vi "Mapping v10.2.2.vi"(5 "Simulate Spectra":bool, 7 "Simulate Drive":bool, 11 "Input Parameters":T9={"CCD3000 Connection"={"Comm Interface"=1, "BUS"=0, "Address"=5, "Com Port"=1}, "Drive Connection Settings"={"Objective GPIB-Port"=4, "Stage GPIB-Port"=4, "Drive Selector"=0, "Drive Velocity (V/s)"=5.0}, "ITC503 Current Values"={"ITC503 Heater"=0.0, "ITC503 Temperature"=0.0, "ITC503 P"=0.0, "ITC503 I"=0.0, "ITC503 D"=0.0, "ITC503 Setpoint"=0.0, "ITC503 Gradient"=0.0, "ITC503 Heater Auto"=FALSE, "ITC503 PID Auto"=FALSE}, "Wavelengths (nm)"=[], "Drive Current Values"={"Voltages"={"Drive X Voltage"=0.0, "Drive Y Voltage"=0.0, "Drive Z Voltage"=0.0}, "Position"={"Drive X Position"=0.0, "Drive Y Position"=0.0, "Drive Z Position"=0.0}}, "iHR Current Values"={"iHR 550 Front Entrance"=0.0, "iHR550 Side Exit"=0.0, "iHR550 Wavelength"=897.9988, "iHR550 Exit Mirror"=2, "iHR550 Grating"="1", "Grating Index"=1}, "Spectra Settings"={"Integration Time"=1.0, "Repetitions"=1, "Mapping Spectra"=TRUE}, "CCD3500 Temperature"=0.0, "Simulate Drive"=FALSE, "Simulate Spectra"=FALSE} {"CCD3500 Temperature" min=10.0 max=160.0 step=0.1 format="%.1f"; "Spectra Settings"."Repetitions" min=1 max=100 step=1; "Spectra Settings"."Integration Time" min=0.5 max=6000.0 step=1.0 format="%.1f"; "iHR Current Values"."iHR550 Exit Mirror" items=["EntranceMirror", "ExitMirror", "Front", "Side"]; "Drive Current Values"."Position"."Drive Z Position" min=-273.0 max=300000.0 step=0.0001 format="%.1f"; "Drive Current Values"."Position"."Drive Y Position" min=-273.0 max=300000.0 step=0.0001 format="%.1f"; "Drive Current Values"."Position"."Drive X Position" min=-273.0 max=300000.0 step=0.0001 format="%.1f"; "Drive Current Values"."Voltages"."Drive Z Voltage" min=-273.0 max=300000.0 step=0.0001 format="%.1f"; "Drive Current Values"."Voltages"."Drive Y Voltage" min=-273.0 max=300000.0 step=0.0001 format="%.1f"; "Drive Current Values"."Voltages"."Drive X Voltage" min=-273.0 max=300000.0 step=0.0001 format="%.1f"; "ITC503 Current Values"."ITC503 Gradient" format="%.2f"; "ITC503 Current Values"."ITC503 Setpoint" min=-273.0 max=300000.0 step=0.0001 format="%.1f"; "ITC503 Current Values"."ITC503 I" format="%_1f"; "ITC503 Current Values"."ITC503 P" format="%_1f"; "ITC503 Current Values"."ITC503 Temperature" min=0.0 max=1645.0 step=1e-05 format="%.2f"; "ITC503 Current Values"."ITC503 Heater" min=0.0 max=100.0 step=0.01 scale=0.0..100.0; "Drive Connection Settings"."Drive Velocity (V/s)" min=10.0 max=160.0 step=0.1 format="%.1f"; "Drive Connection Settings"."Drive Selector" items=["Obj.", "Stage"]; "Drive Connection Settings"."Stage GPIB-Port" min=1 max=20 step=1 format="%#.0f"; "Drive Connection Settings"."Objective GPIB-Port" min=1 max=20 step=1 format="%#.0f"; "CCD3000 Connection"."Comm Interface" items=["RS 232", "GPIB"]}) -> ()   [LabVIEW 2010]
uses:
  ESA-C/TypeDefs/ESA-C Connection Settings.ctl
  TypeDefs/Mapping Spectra Params.ctl
  TypeDefs/Mapping Drive Params.ctl
  ESA-C/TypeDefs/ESA-C Set Positions.ctl
  ESA-C/TypeDefs/ESA-C Current Values.ctl
  iHR550/TypeDefs/iHR Current Values.ctl
  ITC503/TypeDefs/ITC503 Current Values.ctl
  drivers/Horiba Spectrum One 3000V/Lib/CCD_command.llb/Comm Params.ctl
  <vilib>/Utility/miscctls.llb/LVPointTypeDef.ctl
panel:
  in  "Pause":bool
  out "Current Position":T1 {"Position"."Drive Z Position" min=-273.0 max=300000.0 step=0.0001 format="%.1f"; "Position"."Drive Y Position" min=-273.0 max=300000.0 step=0.0001 format="%.1f"; "Position"."Drive X Position" min=-273.0 max=300000.0 step=0.0001 format="%.1f"; "Voltages"."Drive Z Voltage" min=-273.0 max=300000.0 step=0.0001 format="%.1f"; "Voltages"."Drive Y Voltage" min=-273.0 max=300000.0 step=0.0001 format="%.1f"; "Voltages"."Drive X Voltage" min=-273.0 max=300000.0 step=0.0001 format="%.1f"}
  out "Target Position":T2={"Drive X Set"=10.0, "Drive Y Set"=10.0, "Drive Z Set"=10.0} {"Drive X Set" min=10.0 max=160.0 step=0.1 format="%.1f"; "Drive Z Set" min=10.0 max=160.0 step=0.1 format="%.1f"; "Drive Y Set" min=10.0 max=160.0 step=0.1 format="%.1f"}
  out "Progress":u8(slide) max=10 scale=0.0..100.0
  out "Objective Running":bool caption="Obj."
  out "CCD Running":bool caption="CCD"
  in  "Save Map":bool
  in  "CCD3000 Current Rep.":string="0/0"
  in  "Spectra Params":T3={"Integration Time"=10.0, "Repetitions"=10, "Mapping Spectra"=TRUE} {"Repetitions" min=1 max=100 step=1; "Integration Time" min=0.5 max=6000.0 step=1.0 format="%.1f"}
  in  "Drive Settings":T4={"Objective GPIB-Port"=4, "Stage GPIB-Port"=4, "Drive Selector"=0, "Drive Velocity (V/s)"=5.0} {"Drive Velocity (V/s)" min=10.0 max=160.0 step=0.1 format="%.1f"; "Drive Selector" items=["Obj.", "Stage"]; "Stage GPIB-Port" min=1 max=20 step=1 format="%#.0f"; "Objective GPIB-Port" min=1 max=20 step=1 format="%#.0f"}
  in  "Z Position":dbl caption="Z (µm)" min=0.0 max=100.0 step=0.1 format="%.1f"
  in  "Mapping Params":T5={"X Start Position"=0.0, "X Stop Position"=10.0, "Y Start Position"=0.0, "Y Stop Position"=10.0, "Step Size"=1.0} {"Step Size" min=0.1 max=30.0 step=0.1 format="%.1f"; "Y Stop Position" min=0.0 max=30.0 step=0.1 format="%.1f"; "Y Start Position" min=0.0 max=30.0 step=0.1 format="%.1f"; "X Stop Position" min=0.0 max=30.0 step=0.1 format="%.1f"; "X Start Position" min=0.0 max=30.0 step=0.1 format="%.1f"}
  in  "Exit":bool
  out "Measuring":bool
  in  "Start":bool
  out "Filename":string
  out "Full Data":dbl[][](array[numeric])
  in  "CCD3500V Connection":T10={"Comm Interface"=1, "BUS"=0, "Address"=5, "Com Port"=0}
  out "Live Data":dbl[][](array[numeric])
  in  "ITC503 Current Values":T7 {"ITC503 Gradient" format="%.2f"; "ITC503 Setpoint" min=-273.0 max=300000.0 step=0.0001 format="%.1f"; "ITC503 I" format="%_1f"; "ITC503 P" format="%_1f"; "ITC503 Temperature" min=0.0 max=1645.0 step=1e-05 format="%.2f"; "ITC503 Heater" min=0.0 max=100.0 step=0.01 scale=0.0..100.0}
  in  "iHR Current Values":T8={"iHR 550 Front Entrance"=0.0, "iHR550 Side Exit"=0.0, "iHR550 Wavelength"=897.9988, "iHR550 Exit Mirror"=2, "iHR550 Grating"="1", "Grating Index"=1} {"iHR550 Exit Mirror" items=["EntranceMirror", "ExitMirror", "Front", "Side"]}
  in  "CCD3500 Temperature":dbl caption="Temp. (°C)" min=10.0 max=160.0 step=0.1 format="%.1f"
  in  "Wavelengths (nm)":dbl[](array[numeric])
  # "Status"
  # "Active"
  # "Target"
  # "Current"
  # "Spectral"
  # "Spectral / Video Mapping"
  # "Parameters"
  # "GPIB"
  # "Mapping"
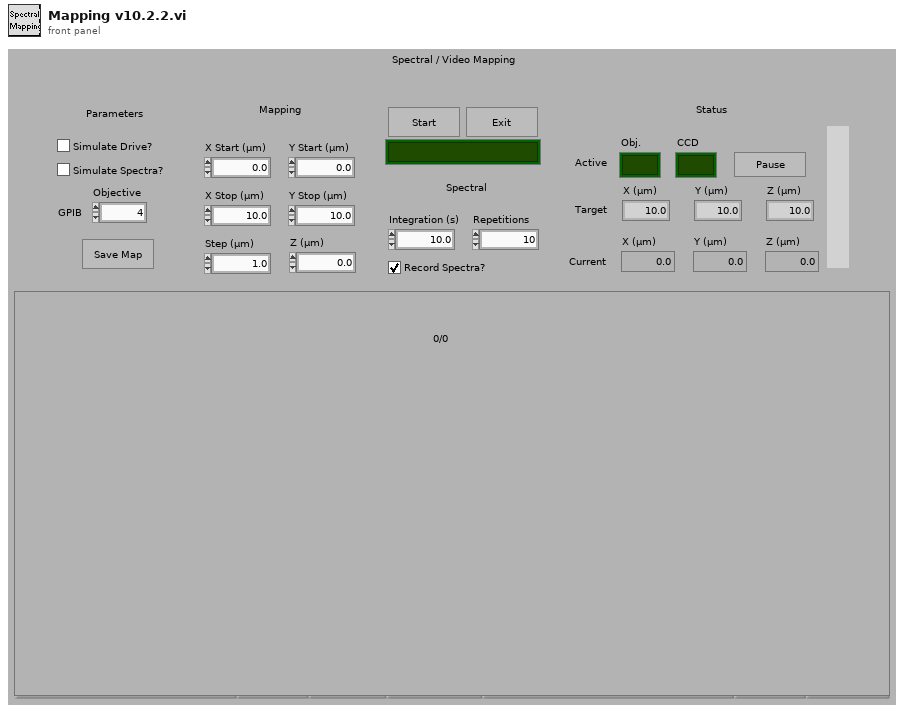
[diagram p1: front panel]
types:
  T1 = typedef "ESA-C Current Values.ctl" = cluster{"Voltages":cluster{"Drive X Voltage":dbl, "Drive Y Voltage":dbl, "Drive Z Voltage":dbl}, "Position":cluster{"Drive X Position":dbl, "Drive Y Position":dbl, "Drive Z Position":dbl}}
  T2 = typedef "ESA-C Set Positions.ctl" = cluster{"Drive X Set":dbl, "Drive Y Set":dbl, "Drive Z Set":dbl}
  T3 = typedef "Mapping Spectra Params.ctl" = cluster{"Integration Time":dbl, "Repetitions":u16, "Mapping Spectra":bool}
  T4 = typedef "ESA-C Connection Settings.ctl" = cluster{"Objective GPIB-Port":i32, "Stage GPIB-Port":i32, "Drive Selector":u16, "Drive Velocity (V/s)":dbl}
  T5 = typedef "Mapping Drive Params.ctl" = cluster{"X Start Position":dbl, "X Stop Position":dbl, "Y Start Position":dbl, "Y Stop Position":dbl, "Step Size":dbl}
  T6 = typedef "Comm Params.ctl" = cluster{"Comm Interface":u16, "BUS":i16, "Address":i16, "Com Port":i32}
  T7 = typedef "ITC503 Current Values.ctl" = cluster{"ITC503 Heater":dbl, "ITC503 Temperature":dbl, "ITC503 P":dbl, "ITC503 I":dbl, "ITC503 D":dbl, "ITC503 Setpoint":dbl, "ITC503 Gradient":dbl, "ITC503 Heater Auto":bool, "ITC503 PID Auto":bool}
  T8 = typedef "iHR Current Values.ctl" = cluster{"iHR 550 Front Entrance":dbl, "iHR550 Side Exit":dbl, "iHR550 Wavelength":dbl, "iHR550 Exit Mirror":i32, "iHR550 Grating":string, "Grating Index":i32}
  T9 = cluster{"CCD3000 Connection":T6, "Drive Connection Settings":T4, "ITC503 Current Values":T7, "Wavelengths (nm)":dbl[], "Drive Current Values":T1, "iHR Current Values":T8, "Spectra Settings":T3, "CCD3500 Temperature":dbl, "Simulate Drive":bool, "Simulate Spectra":bool}
  T10 = cluster{"Comm Interface":u16, "BUS":i16, "Address":i16, "Com Port":i32}
  T11 = cluster{"CCD3000 Connection":T6, "Drive Connection Settings":T4, "ITC503 Current Values":T7, "Wavelengths (nm)":dbl[], "Drive Current Values":T1, "iHR Current Values":T8, "Spectra Settings":T3, "CCD3500 Temperature":dbl, "Simulate Drive 2":bool, "Simulate Spectra 2":bool}
  T12 = typedef "LVPointTypeDef.ctl" = cluster{"Horizontal":i16, "Vertical":i16}
  T13 = typedef "NPC3SG Set Positions.ctl" = cluster{"Drive X Set":dbl, "Drive Y Set":dbl, "Drive Z Set":dbl}
  T14 = cluster{"Intensities":dbl[], "Wavelengths":dbl[]}[]
  T15 = cluster{"Intensities":dbl[], "Wavelengths":dbl[]}
  T16 = enum32{"invalid app kind", "Development System", "Run Time System", "Student Edition", "Embedded LabVIEW", "Evaluation", "Custom"}
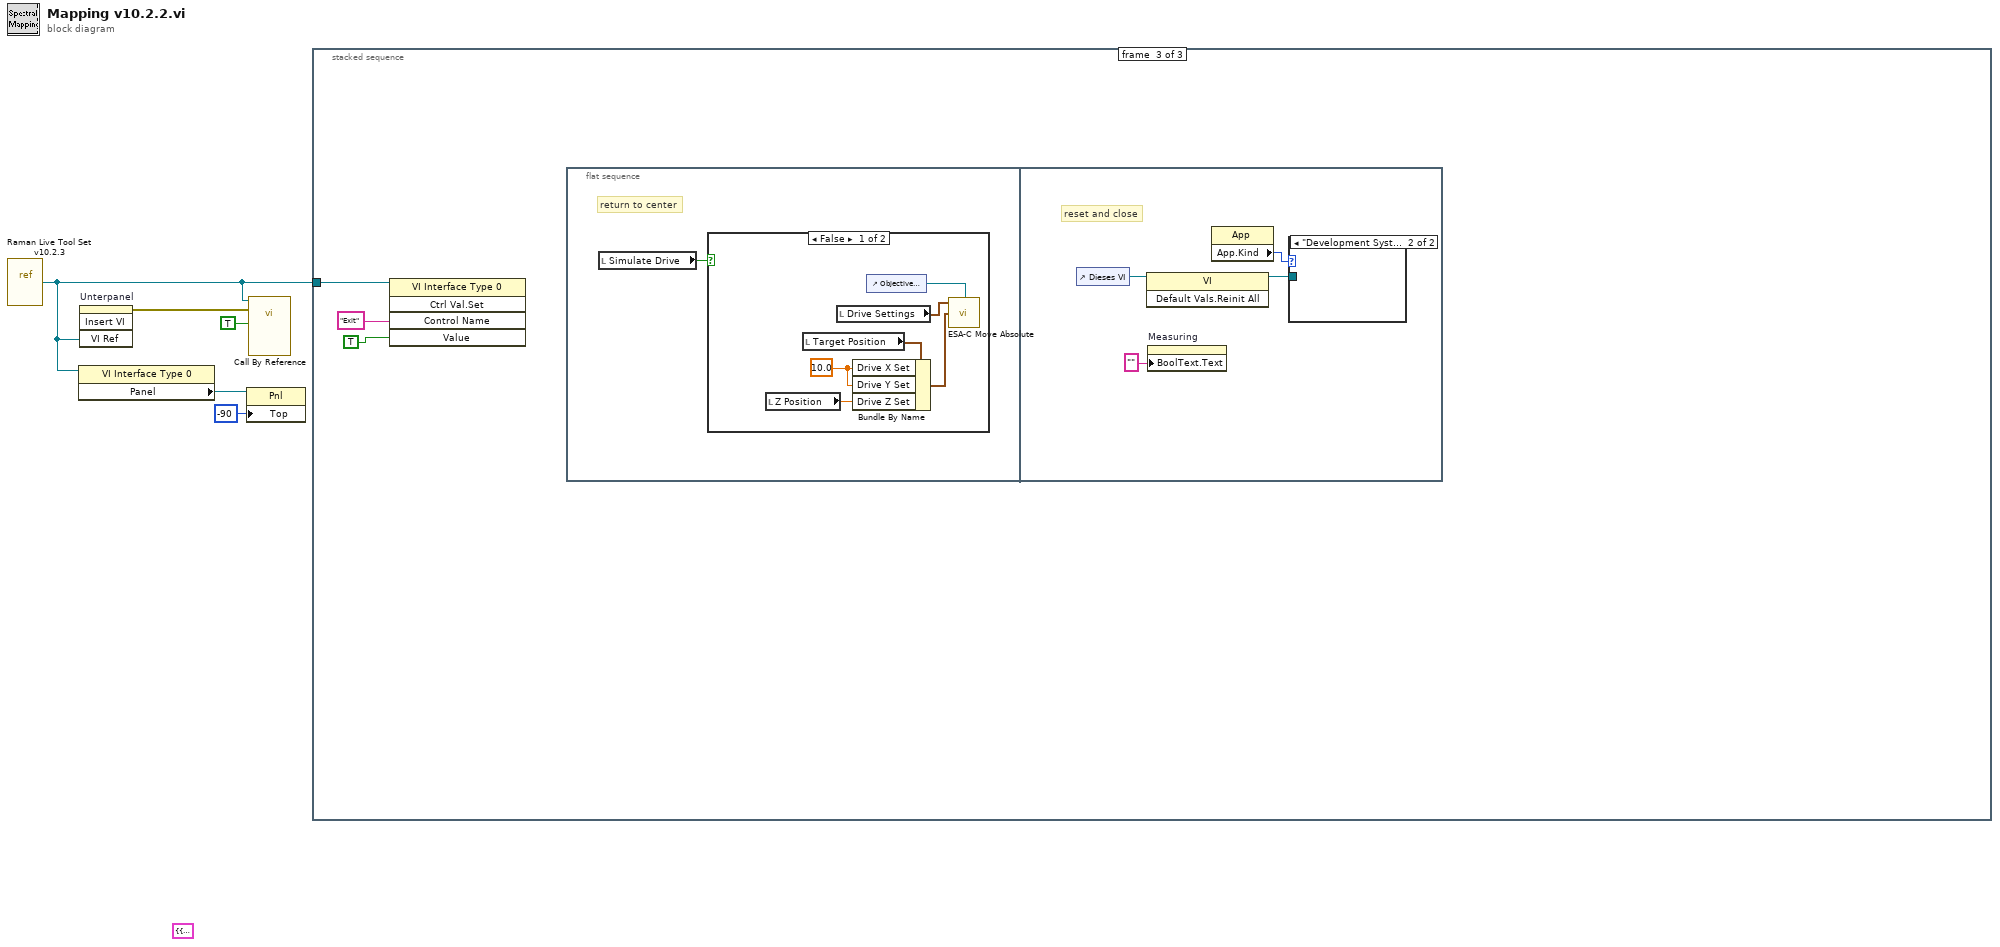
[diagram p0: block diagram]
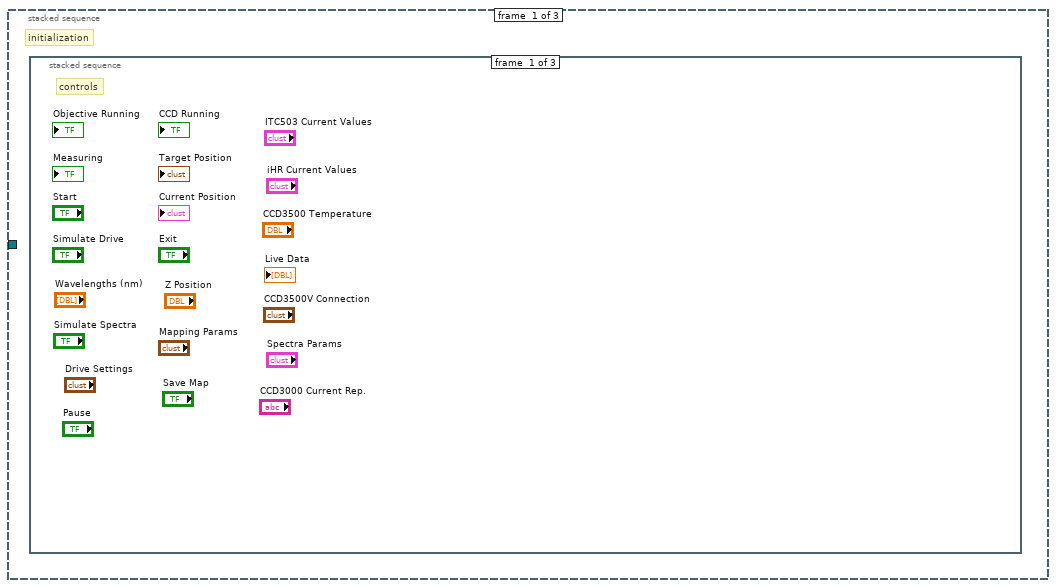
[diagram p2: hidden frame]
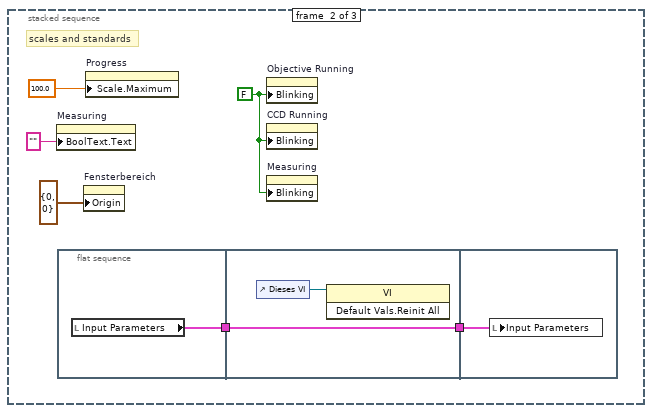
[diagram p3: hidden frame]
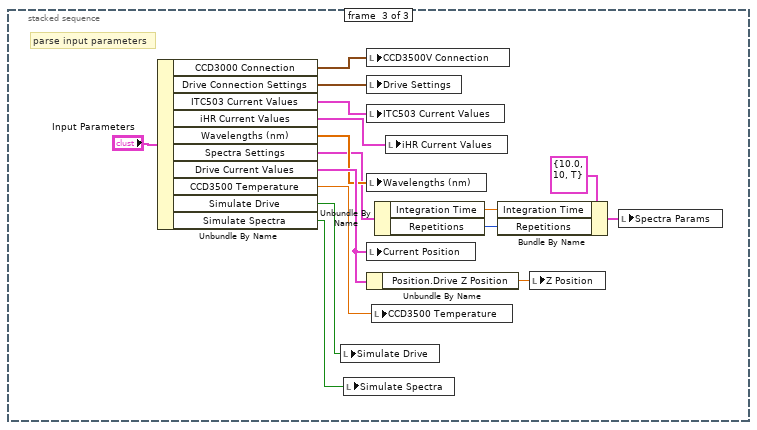
[diagram p4: hidden frame]
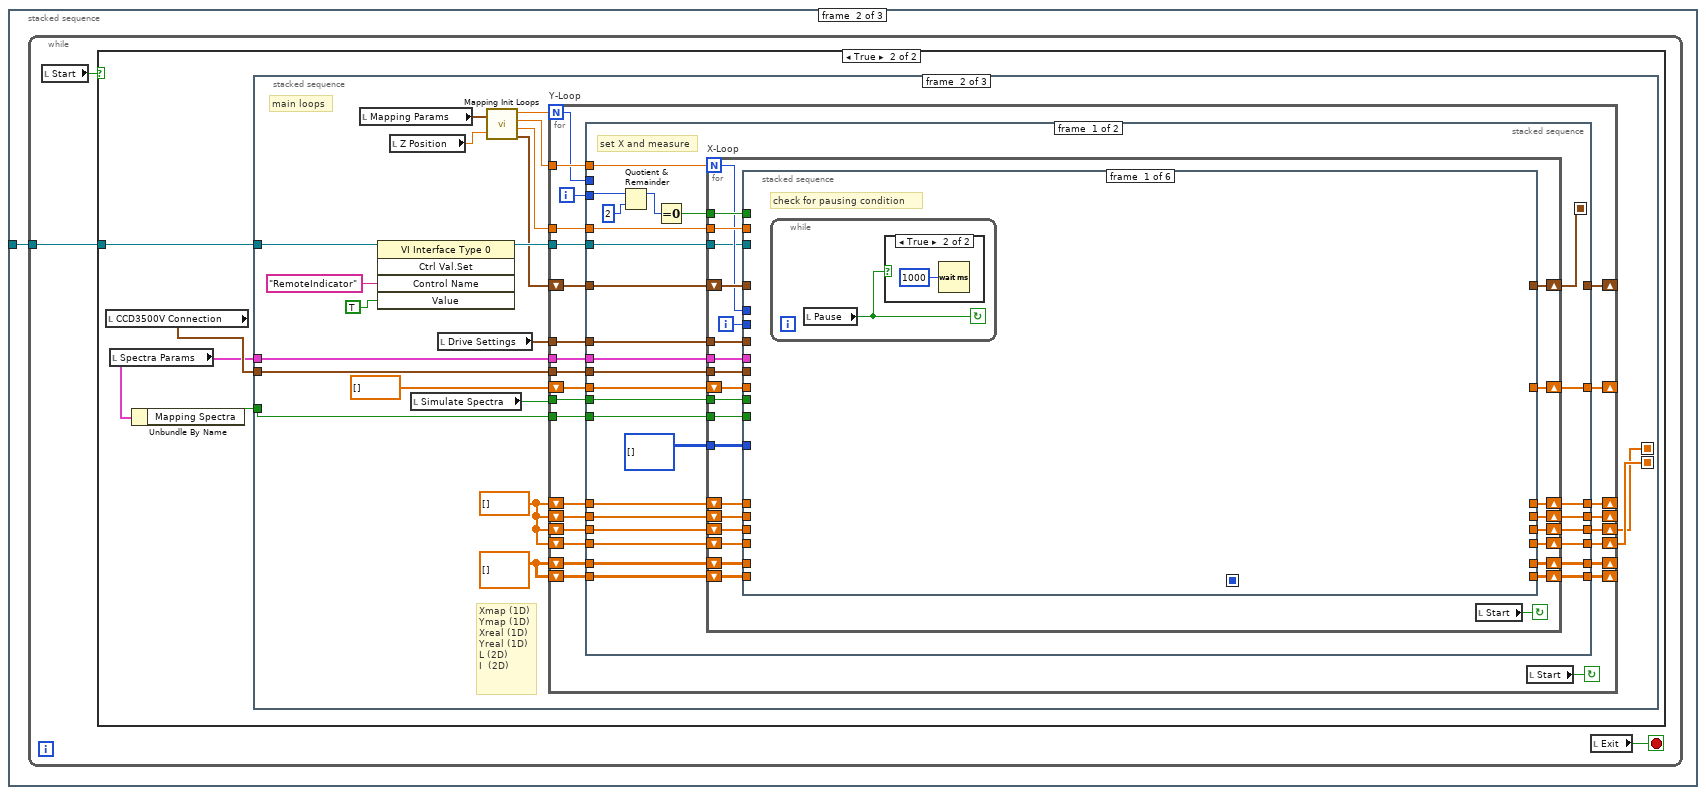
[diagram p5: hidden frame]
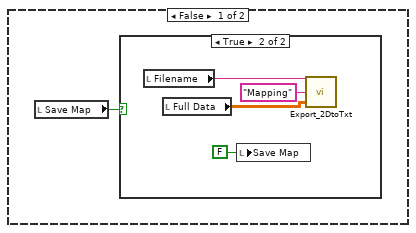
[diagram p6: hidden frame]
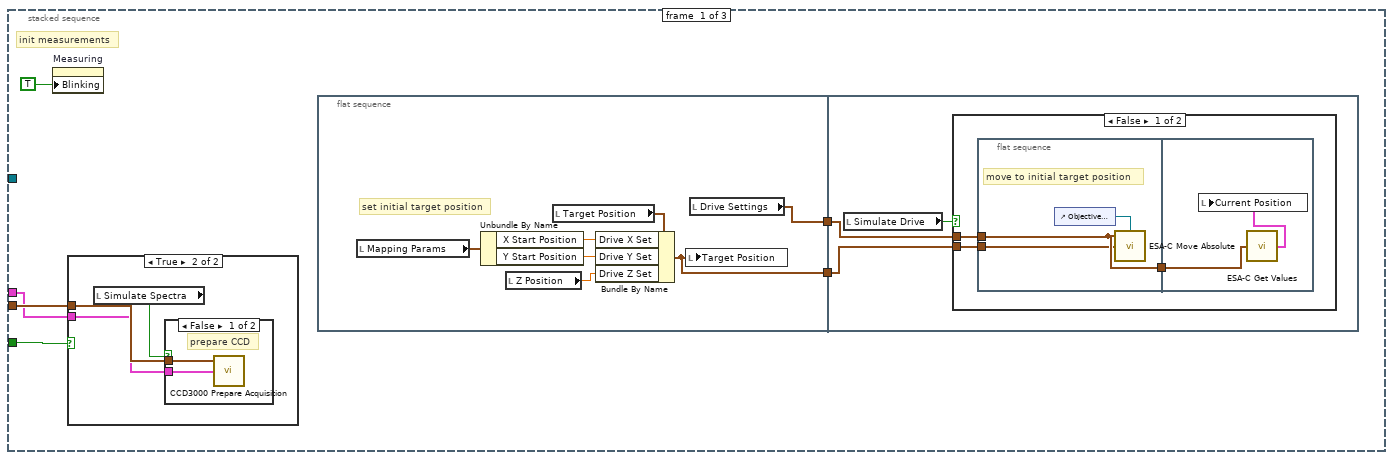
[diagram p8: hidden frame]
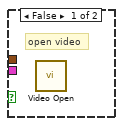
[diagram p10: hidden frame]
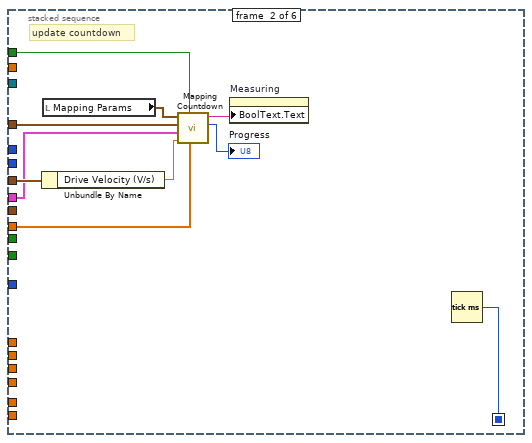
[diagram p13: hidden frame]
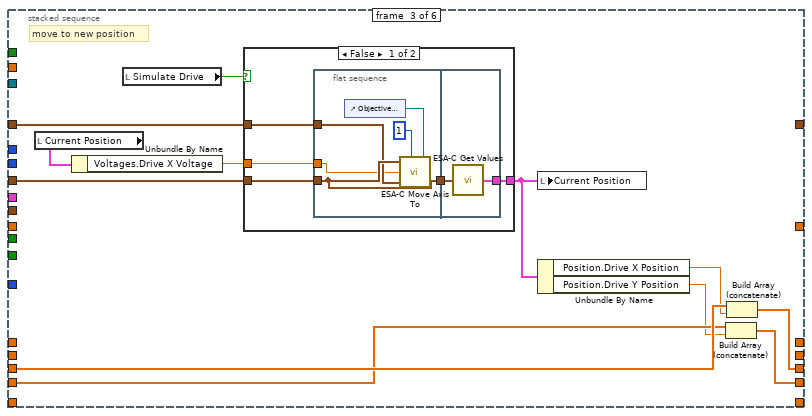
[diagram p14: hidden frame]
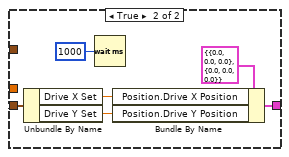
[diagram p15: hidden frame]
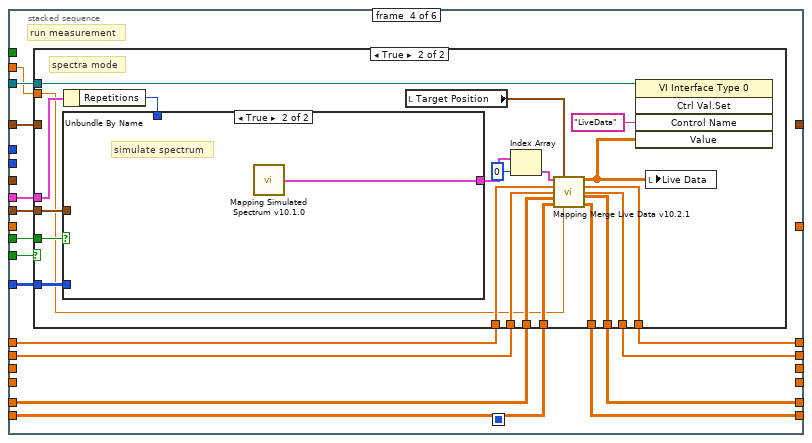
[diagram p16: hidden frame]
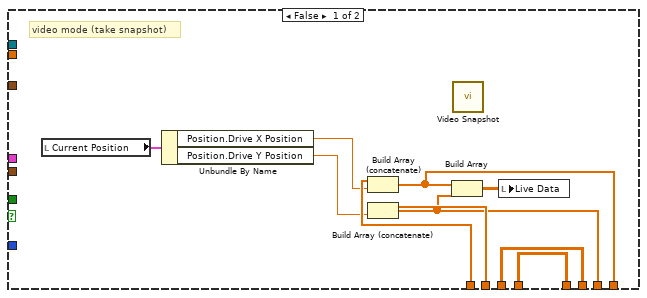
[diagram p17: hidden frame]
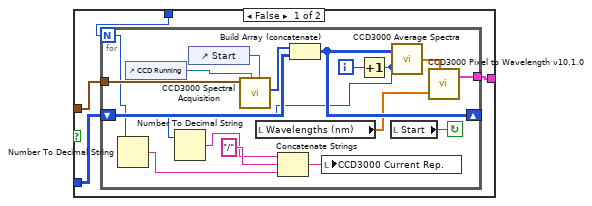
[diagram p18: hidden frame]
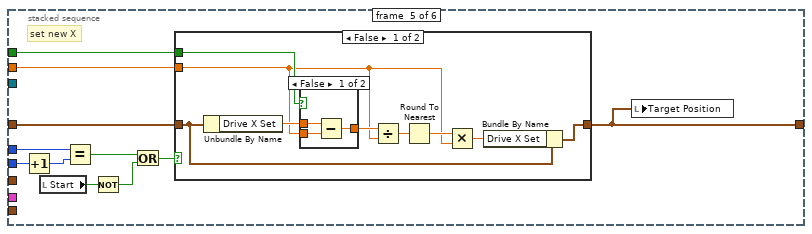
[diagram p19: hidden frame]
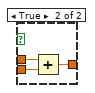
[diagram p20: hidden frame]
diagram:
  (unwired) T11 {"CCD3000 Connection"={"Comm Interface"=1, "BUS"=0, "Address"=5, "Com Port"=1}, "Drive Connection Settings"={"Objective GPIB-Port"=4, "Stage GPIB-Port"=4, "Drive Selector"=0, "Drive Velocity (V/s)"=5.0}, "ITC503 Current Values"={"ITC503 Heater"=0.0, "ITC503 Temperature"=0.0, "ITC503 P"=0.0, "ITC503 I"=0.0, "ITC503 D"=0.0, "ITC503 Setpoint"=0.0, "ITC503 Gradient"=0.0, "ITC503 Heater Auto"=FALSE, "ITC503 PID Auto"=FALSE}, "Wavelengths (nm)"=[], "Drive Current Values"={"Voltages"={"Drive X Voltage"=0.0, "Drive Y Voltage"=0.0, "Drive Z Voltage"=0.0}, "Position"={"Drive X Position"=0.0, "Drive Y Position"=0.0, "Drive Z Position"=0.0}}, "iHR Current Values"={"iHR 550 Front Entrance"=0.0, "iHR550 Side Exit"=0.0, "iHR550 Wavelength"=897.9988, "iHR550 Exit Mirror"=2, "iHR550 Grating"="1", "Grating Index"=1}, "Spectra Settings"={"Integration Time"=1.0, "Repetitions"=1, "Mapping Spectra"=TRUE}, "CCD3500 Temperature"=0.0, "Simulate Drive 2"=FALSE, "Simulate Spectra 2"=FALSE} ("Input Parameters")
  n1 = vi-ref "Raman Live Tool Set v10.2.3.vi"() -> (w3:refnum<vi>)
  n2 = property class="VI Interface Type 0"(reference=w3) -> ("Panel"=w2:refnum<vi>)  [unwired: 1 in, 2 out]
  n3 = invoke on="Unterpanel" class="Unterpanel" method="Insert VI"("VI Ref"=w3) -> (error out=w5:errorcluster)  [unwired: 3 in, 3 out]
  n4 = property class="Pnl"(reference=w2, "Top"=-90 ("Position:Oben")) -> ()  [unwired: 1 in, 2 out]
  n5 = call-by-ref "?"(reference=w3, error in=w5, "RemoteIndicator"=TRUE) -> ()  [unwired: 3 in, 2 out]
  n6 = stacked-sequence {
    tunnel: w3 -> [_ w32 w390]
    frame #0 {
      # "initialization"
      n7 = stacked-sequence {
        frame #0 {
          # "controls"
        }
        frame #1 {
          w9 = FALSE ("Blinkend")
          # "scales and standards"
          n8 = property on="Measuring" class="Bool (strict)"("BoolText.Text"="" ("Boolescher Text.Text")) -> ()  [unwired: 2 in, 2 out]
          n9 = flat-sequence {
            tunnel: [w12] -> w6
            tunnel: [w13] -> w7
            tunnel: w6 -> [w13]
            tunnel: w7 -> [w15]
            frame #0 {
              n10 = local read "Input Parameters"() -> (w12:T9)
            }
            frame #1 {
              n11 = control-ref of="Dieses VI"() -> (w14:refnum<vi>)
              n12 = invoke class="VI" method="Default Vals.Reinit All"(reference=w14) -> ()  [unwired: 2 in, 3 out]
            }
            frame #2 {
              n13 = local write "Input Parameters"(w15) -> ()
            }
          }
          n14 = property on="Fensterbereich" class="Pane"("Origin"=T12 {"Horizontal"=0, "Vertical"=0}) -> ()  [unwired: 2 in, 2 out]
          n15 = property on="Progress" class="Slide (strict)"("Scale.Maximum"=100.0 ("Skalierung.Bereich:Maximum")) -> ()  [unwired: 2 in, 2 out]
          n16 = property on="Objective Running" class="Bool (strict)"("Blinking"=w9) -> ()  [unwired: 2 in, 2 out]
          n17 = property on="CCD Running" class="Bool (strict)"("Blinking"=w9) -> ()  [unwired: 2 in, 2 out]
          n18 = property on="Measuring" class="Bool (strict)"("Blinking"=w9) -> ()  [unwired: 2 in, 2 out]
        }
        frame #2 {
          # "parse input parameters"
          n19 = Unbundle By Name("Input Parameters") -> ("CCD3000 Connection"=w28:T6, "Drive Connection Settings"=w29:T4, "ITC503 Current Values"=w30:T7, "iHR Current Values"=w19:T8, "Wavelengths (nm)"=w27:dbl[], "Spectra Settings"=w25:T3, "Drive Current Values"=w31:T1, "CCD3500 Temperature"=w20:dbl, "Simulate Drive"=w17:bool, "Simulate Spectra"=w16:bool)
          n20 = local write "Simulate Drive"(w17) -> ()
          n21 = local write "Simulate Spectra"(w16) -> ()
          n22 = local write "CCD3500V Connection"(w28) -> ()
          n23 = local write "Drive Settings"(w29) -> ()
          n24 = local write "ITC503 Current Values"(w30) -> ()
          n25 = local write "Wavelengths (nm)"(w27) -> ()
          n26 = local write "Current Position"(w31) -> ()
          n27 = Unbundle By Name(w31) -> ("Position.Drive Z Position"=w26:dbl)
          n28 = local write "CCD3500 Temperature"(w20) -> ()
          n29 = Unbundle By Name(w25) -> ("Integration Time"=w23:dbl, "Repetitions"=w22:u16)
          n30 = local write "iHR Current Values"(w19) -> ()
          n31 = Bundle By Name(cluster=T3 {"Integration Time"=10.0, "Repetitions"=10, "Mapping Spectra"=TRUE} ("Mapping Spectra Settings"), "Integration Time"=w23, "Repetitions"=w22) -> (w21:T3)
          n32 = local write "Z Position"(w26) -> ()
          n33 = local write "Spectra Params"(w21) -> ()
        }
      }
    }
    frame #1 {
      n34 = while {
        tunnel: w32 -> [w35]
        stop <- w34 stop-if-true
        n35 = local read "Start"() -> (w33:bool)
        n36 = case shown="True" w33 {
          tunnel: w35 -> [_ w44]
          frame False {
            n37 = local read "Save Map"() -> (w36:bool)
            n38 = case shown="True" w36 {
              frame False {
              }
              frame True {
                n39 = local read "Filename"() -> (w39:string)
                n40 = local read "Full Data"() -> (w37:dbl[][])
                n41 = local write "Save Map"(FALSE ("Save Map")) -> ()
                n42 = call "Export_2DtoTxt.vi"("Data (2D)"=w37, "Export Type"="Mapping", "Filename"=w39) -> ()  [unwired: 3 in]
              }
            }
          }
          frame True {
            n43 = local read "CCD3500V Connection"() -> (w42:T10)
            n44 = local read "Spectra Params"() -> (w41:T3)
            n45 = Unbundle By Name(w41) -> ("Mapping Spectra"=w43:bool)
            n46 = stacked-sequence {
              seq-local: [_ w74 _] -> [_ _ w358]
              seq-local: [_ w75 _] -> [_ _ w357]
              tunnel: w44 -> [_ w85 _]
              tunnel: w43 -> [w49 w84 w359]
              tunnel: w41 -> [w47 w82 _]
              tunnel: w42 -> [w48 w81 _]
              frame #0 {
                # "init measurements"
                n47 = property on="Measuring" class="Bool (strict)"("Blinking"=TRUE ("Blinkend")) -> ()  [unwired: 2 in, 2 out]
                n48 = case shown="True" w49 {
                  tunnel: w48 -> [_ w71]
                  tunnel: w47 -> [_ w70]
                  frame False {
                    # "open video"
                    n49 = call "Video Open.vi"() -> ()  [unwired: 11 in, 1 out]
                  }
                  frame True {
                    n50 = local read "Simulate Spectra"() -> (w69:bool)
                    n51 = case shown="False" w69 {
                      tunnel: w71 -> [w73 _]
                      tunnel: w70 -> [w72 _]
                      frame False {
                        # "prepare CCD"
                        n52 = call "CCD3000 Prepare Acquisition.vi"("Mapping Spectra Settings"=w72, "Comm Params"=w73) -> ()  [unwired: 4 in]
                      }
                      frame True {
                      }
                    }
                  }
                }
                n53 = flat-sequence {
                  tunnel: [w52] -> w46
                  tunnel: [w51] -> w45
                  tunnel: w46 -> [w58]
                  tunnel: w45 -> [w59]
                  frame #0 {
                    # "set initial target position"
                    n54 = local read "Mapping Params"() -> (w57:T5)
                    n55 = Unbundle By Name(w57) -> ("X Start Position"=w55:dbl, "Y Start Position"=w54:dbl)
                    n56 = local read "Z Position"() -> (w53:dbl)
                    n57 = local read "Target Position"() -> (w56:T2)
                    n58 = Bundle By Name(cluster=w56, "Drive X Set"=w55, "Drive Y Set"=w54, "Drive Z Set"=w53) -> (w52:T2)
                    n59 = local write "Target Position"(w52) -> ()
                    n60 = local read "Drive Settings"() -> (w51:T4)
                  }
                  frame #1 {
                    n61 = local read "Simulate Drive"() -> (w60:bool)
                    n62 = case shown="False" w60 {
                      tunnel: w59 -> [w63 _]
                      tunnel: w58 -> [w61 _]
                      frame False {
                        n63 = flat-sequence {
                          tunnel: w63 -> [w65]
                          tunnel: [w65] -> w62
                          tunnel: w61 -> [w64]
                          tunnel: w62 -> [w68]
                          frame #0 {
                            # "move to initial target position"
                            n64 = control-ref of="Objective Running"() -> (w66:refnum<vi>)
                            n65 = call "ESA-C Move Absolute.vi"("Running"=w66, "Drive New Abs. Positions"=w64, "Drive Connection Settings"=w65) -> ()  [unwired: 2 in]
                          }
                          frame #1 {
                            n66 = call "ESA-C Get Values.vi"("Drive Connection Settings"=w68) -> ("Drive Current Values"=w67:T1)
                            n67 = local write "Current Position"(w67) -> ()
                          }
                        }
                      }
                      frame True {
                      }
                    }
                  }
                }
              }
              frame #1 {
                w93 = dbl[][] []
                w76 = dbl[] []
                # "main loops"
                # "Xmap (1D)\nYmap (1D)\nXreal (1D)\nYreal (1D)\nL (2D)\nI  (2D)"
                n68 = local read "Mapping Params"() -> (w79:T5)
                n69 = invoke class="VI Interface Type 0" method="Ctrl Val.Set"(reference=w85, "Control Name"="RemoteIndicator" ("Elementname"), "Value"=TRUE) -> (reference out=w87:refnum<vi>)  [unwired: 2 in, 4 out]
                n70 = local read "Z Position"() -> (w78:dbl)
                n71 = local read "Simulate Spectra"() -> (w77:bool)
                n72 = local read "Drive Settings"() -> (w80:T4)
                n73 = call "Mapping Init Loops.vi"("Z Position"=w78, "Mapping Params"=w79) -> ("Start Positions"=w86:T13, "Step Size"=w88:dbl, "X Steps"=w89:dbl, "Y Steps"=w90:dbl)
                n74 = for "Y-Loop" {
                  N: w90 -> [w106]
                  tunnel: w89 -> [w119]
                  tunnel: w88 -> [w118]
                  shift-right: [w104] -> _
                  shift-left: w86 -> [w105]
                  shift-right: [w110] -> _
                  shift-left: w93 -> [w114]
                  shift-right: [w111] -> _
                  shift-left: w93 -> [w115]
                  shift-right: [w113] -> _
                  shift-left: w76 -> [w117]
                  shift-right: [w112] -> _
                  shift-left: w76 -> [w116]
                  tunnel: w87 -> [w108]
                  tunnel: w77 -> [w107]
                  tunnel: w80 -> [w103]
                  tunnel: w84 -> [w102]
                  tunnel: w82 -> [w101]
                  shift-right: [w99] -> _
                  shift-left: dbl[] [] -> [w100]
                  tunnel: w81 -> [w98]
                  shift-right: [w95] -> w75
                  shift-left: w76 -> [w96]
                  shift-right: [w94] -> w74
                  shift-left: w76 -> [w97]
                  i -> [w109]
                  stop <- w120 continue-if-true
                  n75 = stacked-sequence {
                    seq-local: [w133 _] -> [_ w330]
                    tunnel: w119 -> [w149 _]
                    tunnel: w118 -> [w148 w331]
                    tunnel: w117 -> [w147 _]
                    tunnel: w116 -> [w146 _]
                    tunnel: w115 -> [w145 _]
                    tunnel: w114 -> [w144 _]
                    tunnel: [w143 _] -> w113
                    tunnel: [w142 _] -> w112
                    tunnel: [w141 _] -> w111
                    tunnel: [w140 _] -> w110
                    tunnel: w109 -> [w137 w334]
                    tunnel: w108 -> [w135 _]
                    tunnel: w107 -> [w134 _]
                    tunnel: w106 -> [_ w332]
                    tunnel: w105 -> [w132 _]
                    tunnel: [_ w328] -> w104
                    tunnel: w103 -> [w131 w329]
                    tunnel: w102 -> [w130 _]
                    tunnel: w101 -> [w129 _]
                    tunnel: w100 -> [w128 _]
                    tunnel: [w127 _] -> w99
                    tunnel: w98 -> [w126 _]
                    tunnel: w97 -> [w124 _]
                    tunnel: w96 -> [w123 _]
                    tunnel: [w122 _] -> w95
                    tunnel: [w121 _] -> w94
                    frame #0 {
                      # "set X and measure"
                      n76 = Quotient & Remainder(x=w137, y=2) -> (x-y*floor(x/y)=w138:i32)  [unwired: 1 out]
                      n77 = Equal To 0?(x=w138) -> (x = 0?=w136:bool)
                      n78 = for "X-Loop" {
                        N: w149 -> [w163]
                        tunnel: w148 -> [w175]
                        shift-right: [w174] -> w133
                        shift-left: w132 -> [w176]
                        shift-right: [w169] -> w143
                        shift-left: w147 -> [w173]
                        shift-right: [w168] -> w142
                        shift-left: w146 -> [w172]
                        shift-right: [w166] -> w141
                        shift-left: w145 -> [w171]
                        shift-right: [w167] -> w140
                        shift-left: w144 -> [w170]
                        tunnel: w136 -> [w165]
                        tunnel: w135 -> [w162]
                        tunnel: w134 -> [w161]
                        tunnel: w131 -> [w160]
                        tunnel: w130 -> [w159]
                        tunnel: w129 -> [w158]
                        shift-right: [w157] -> w127
                        shift-left: w128 -> [w156]
                        tunnel: w126 -> [w155]
                        tunnel: u16[][] [] -> [w154]
                        shift-right: [w150] -> w121
                        shift-left: w124 -> [w153]
                        shift-right: [w151] -> w122
                        shift-left: w123 -> [w152]
                        i -> [w164]
                        stop <- w177 continue-if-true
                        n79 = stacked-sequence {
                          seq-local: [_ w180 _ _ _ _] -> [_ _ _ _ _ w319]
                          tunnel: w176 -> [_ w185 w201 w235 w296 _]
                          tunnel: w175 -> [_ _ _ w220 w294 _]
                          tunnel: [_ _ _ _ w293 _] -> w174
                          tunnel: w173 -> [_ _ _ w234 _ _]
                          tunnel: w172 -> [_ _ _ w233 _ _]
                          tunnel: w171 -> [_ _ _ w231 _ _]
                          tunnel: w170 -> [_ _ _ w232 _ _]
                          tunnel: [_ _ _ w230 _ _] -> w169
                          tunnel: [_ _ _ w229 _ _] -> w168
                          tunnel: [_ _ _ w228 _ _] -> w167
                          tunnel: [_ _ _ w227 _ _] -> w166
                          tunnel: w165 -> [_ w186 _ _ w295 _]
                          tunnel: w164 -> [_ _ _ _ w299 _]
                          tunnel: w163 -> [_ _ _ _ w297 _]
                          tunnel: w162 -> [_ _ _ w226 _ _]
                          tunnel: w161 -> [_ _ _ w225 _ _]
                          tunnel: w160 -> [_ w183 w199 _ _ _]
                          tunnel: w159 -> [_ _ _ w224 _ _]
                          tunnel: w158 -> [_ w182 _ w222 _ _]
                          tunnel: [_ _ _ _ _ w316] -> w157
                          tunnel: w156 -> [_ w181 _ _ _ w318]
                          tunnel: w155 -> [_ _ _ w223 _ _]
                          tunnel: w154 -> [_ _ _ w221 _ _]
                          tunnel: w153 -> [_ _ w195 _ _ _]
                          tunnel: w152 -> [_ _ w194 _ _ _]
                          tunnel: [_ _ w191 _ _ _] -> w151
                          tunnel: [_ _ w190 _ _ _] -> w150
                          frame #0 {
                            # "check for pausing condition"
                            n80 = while {
                              stop <- w178 continue-if-true
                              n81 = local read "Pause"() -> (w178:bool)
                              n82 = case shown="True" w178 {
                                frame False {
                                }
                                frame True {
                                n83 = Wait (ms)(milliseconds to wait=u32 1000) -> ()  [unwired: 1 out]
                                }
                              }
                            }
                          }
                          frame #1 {
                            # "update countdown"
                            n84 = Unbundle By Name(w183) -> ("Drive Velocity (V/s)"=w184:dbl)
                            n85 = local read "Mapping Params"() -> (w189:T5)
                            n86 = call "Mapping Countdown.vi"("Execution Times (s)"=w181, "Forward?"=w186, "Drive Velocity"=w184, "Mapping Spectra Settings"=w182, "Drive New Abs. Positions"=w185, "Mapping Drive Parameters"=w189) -> ("Progress"=→"Progress":i16, "Time String"=w187:string)  [unwired: 4 in]
                            n87 = property on="Measuring" class="Bool (strict)"("BoolText.Text"=w187) -> ()  [unwired: 2 in, 2 out]
                            n88 = Tick Count (ms)() -> (millisecond timer value=w180:u32)
                          }
                          frame #2 {
                            # "move to new position"
                            n89 = local read "Current Position"() -> (w198:T1)
                            n90 = Unbundle By Name(w198) -> ("Voltages.Drive X Voltage"=w197:dbl)
                            n91 = local read "Simulate Drive"() -> (w200:bool)
                            n92 = case shown="False" w200 {
                              tunnel: w201 -> [w205 w218]
                              tunnel: [w204 w215] -> w196
                              tunnel: w199 -> [w203 _]
                              tunnel: w197 -> [w202 _]
                              frame False {
                                n93 = flat-sequence {
                                tunnel: w205 -> [w210]
                                tunnel: [w211] -> w206
                                tunnel: w203 -> [w211]
                                tunnel: w202 -> [w207]
                                tunnel: w206 -> [w213]
                                tunnel: [w212] -> w204
                                frame #0 {
                                n94 = control-ref of="Objective Running"() -> (w208:refnum<vi>)
                                n95 = call "ESA-C Move Axis To.vi"("Drive Connection Settings"=w211, "Axis"=1, "Current Voltage (V)"=w207, "Drive New Abs. Positions"=w210, "Running"=w208) -> ()  [unwired: 2 in]
                                }
                                frame #1 {
                                n96 = call "ESA-C Get Values.vi"("Drive Connection Settings"=w213) -> ("Drive Current Values"=w212:T1)
                                }
                                }
                              }
                              frame True {
                                n97 = Unbundle By Name(w218) -> ("Drive X Set"=w219:dbl, "Drive Y Set"=w216:dbl)
                                n98 = Wait (ms)(milliseconds to wait=u32 1000 ("Zu wartende ms")) -> ()  [unwired: 1 out]
                                n99 = Bundle By Name(cluster=T1 {"Voltages"={"Drive X Voltage"=0.0, "Drive Y Voltage"=0.0, "Drive Z Voltage"=0.0}, "Position"={"Drive X Position"=0.0, "Drive Y Position"=0.0, "Drive Z Position"=0.0}} ("Drive Current Values"), "Position.Drive X Position"=w219, "Position.Drive Y Position"=w216) -> (w215:T1)
                              }
                            }
                            n100 = local write "Current Position"(w196) -> ()
                            n101 = Unbundle By Name(w196) -> ("Position.Drive X Position"=w193:dbl, "Position.Drive Y Position"=w192:dbl)
                            n102 = Build Array (concatenate)(w194, w192) -> (w191:dbl[])
                            n103 = Build Array (concatenate)(w195, w193) -> (w190:dbl[])
                          }
                          frame #3 {
                            # "run measurement"
                            n104 = case shown="True" w224 {
                              tunnel: w235 -> [_ _]
                              tunnel: w234 -> [w242 w263]
                              tunnel: w233 -> [w241 w262]
                              tunnel: w232 -> [w244 w260]
                              tunnel: w231 -> [w245 w261]
                              tunnel: [w239 w257] -> w230
                              tunnel: [w240 w256] -> w229
                              tunnel: [w244 w259] -> w228
                              tunnel: [w245 w258] -> w227
                              tunnel: w226 -> [_ w265]
                              tunnel: w225 -> [_ w264]
                              tunnel: w223 -> [_ w253]
                              tunnel: w222 -> [_ w252]
                              tunnel: w221 -> [_ w250]
                              tunnel: w220 -> [_ w246]
                              frame False {
                                # "video mode (take snapshot)"
                                n105 = local read "Current Position"() -> (w243:T1)
                                n106 = Unbundle By Name(w243) -> ("Position.Drive X Position"=w238:dbl, "Position.Drive Y Position"=w237:dbl)
                                n107 = Build Array (concatenate)(w242, w238) -> (w239:dbl[])
                                n108 = Build Array (concatenate)(w241, w237) -> (w240:dbl[])
                                n109 = Build Array(w239, w240) -> (w236:dbl[][])
                                n110 = call "Video Snapshot.vi"() -> ()  [unwired: 11 in, 1 out]
                                n111 = local write "Live Data"(w236) -> ()
                              }
                              frame True {
                                # "spectra mode"
                                n112 = Unbundle By Name(w252) -> ("Repetitions"=w251:u16)
                                n113 = case shown="True" w264 {
                                tunnel: [w269 w288] -> w249
                                tunnel: w253 -> [w270 _]
                                tunnel: w251 -> [w268 _]
                                tunnel: w250 -> [w267 _]
                                frame False {
                                n114 = for {
                                N: w268 -> [w272]
                                shift-right: [w284] -> _
                                shift-left: w267 -> [w285]
                                tunnel: [w282] -> w269
                                tunnel: w270 -> [w280]
                                i -> [w287]
                                stop <- w279 continue-if-true
                                n115 = Number To Decimal String(number=w272) -> (decimal integer string=w275:string)  [unwired: 1 in]
                                n116 = control-ref of="CCD Running"() -> (w278:refnum<vi>)
                                n117 = control-ref of="Start"() -> (w277:refnum<vi>)
                                n118 = call "CCD3000 Spectral Acquisition.vi"("Acquire"=w277, "Running"=w278, "Comm Params"=w280) -> ("Raw-Spectrum"=w286:u16[])  [unwired: 6 in, 2 out]
                                n119 = local read "Wavelengths (nm)"() -> (w281:dbl[])
                                n120 = Build Array (concatenate)(w286, w285) -> (w284:u16[][])
                                n121 = Increment(x=w287) -> (x+1=w271:i32)
                                n122 = Number To Decimal String(number=w271) -> (decimal integer string=w274:string)  [unwired: 1 in]
                                n123 = Concatenate Strings(w274, "/" ("string"), w275) -> (w273:string)
                                n124 = local write "CCD3000 Current Rep."(w273) -> ()
                                n125 = local read "Start"() -> (w279:bool)
                                n126 = call "CCD3000 Average Spectra.vi"("Repetitions"=w271, "Raw Spectra"=w284) -> ("Raw Spectrum"=w283:dbl[])
                                n127 = call "CCD3000 Pixel to Wavelength v10.1.0.vi"("Wavelengths (nm)"=w281, "Raw Spectrum"=w283) -> ("Spectrum-Cluster"=w282:T14)  [unwired: 1 out]
                                }
                                }
                                frame True {
                                # "simulate spectrum"
                                n128 = call "Mapping Simulated Spectrum v10.1.0.vi"() -> ("Simulated Spectrum"=w288:cluster{i32[], dbl[]}[])
                                }
                                }
                                n129 = local read "Target Position"() -> (w255:T2)
                                n130 = Index Array(array=w249, index=0 ("Index")) -> (element=w248:T15)
                                n131 = call "Mapping Merge Live Data v10.2.1.vi"("New Spectrum"=w248, "Target Position"=w255, "X in (1D)"=w263, "Y in (1D)"=w262, "L in (2D)"=w261, "I in (2D)"=w260, "Step Size"=w246) -> ("Live Data"=w254:dbl[][], "X out (1D)"=w257:dbl[], "Y out (1D)"=w256:dbl[], "L out (2D)"=w258:dbl[][], "I out (2D)"=w259:dbl[][])  [unwired: 4 in]
                                n132 = invoke class="VI Interface Type 0" method="Ctrl Val.Set"(reference=w265, "Control Name"="LiveData" ("Elementname"), "Value"=w254) -> ()  [unwired: 2 in, 5 out]
                                n133 = local write "Live Data"(w254) -> ()
                              }
                            }
                          }
                          frame #4 {
                            # "set new X"
                            n134 = Increment(x=w299) -> (x+1=w298:i32)
                            n135 = local read "Start"() -> (w292:bool)
                            n136 = Equal?(x=w297, y=w298) -> (x = y?=w289:bool)
                            n137 = Not(x=w292) -> (.not. x?=w291:bool)
                            n138 = Or(x=w289, y=w291) -> (x .or. y?=w290:bool)
                            n139 = case shown="False" w290 {
                              tunnel: w296 -> [w307 w315]
                              tunnel: [w306 w315] -> w293
                              tunnel: w295 -> [w305 _]
                              tunnel: w294 -> [w300 _]
                              frame False {
                                n140 = Unbundle By Name(w307) -> ("Drive X Set"=w308:dbl)
                                n141 = case shown="False" w305 {
                                tunnel: w308 -> [w311 w313]
                                tunnel: [w310 w314] -> w301
                                tunnel: w300 -> [w309 w312]
                                frame False {
                                n142 = Subtract(x=w311, y=w309) -> (x-y=w310:dbl)
                                }
                                frame True {
                                n143 = Add(x=w313, y=w312) -> (x+y=w314:dbl)
                                }
                                }
                                n144 = Divide(x=w301, y=w300) -> (x/y=w304:dbl)
                                n145 = Round To Nearest(number=w304) -> (nearest integer value=w303:dbl)
                                n146 = Multiply(x=w303, y=w300) -> (x*y=w302:dbl)
                                n147 = Bundle By Name(cluster=w307, "Drive X Set"=w302) -> (w306:T13)
                              }
                              frame True {
                              }
                            }
                            n148 = local write "Target Position"(w293) -> ()
                          }
                          frame #5 {
                            n149 = Tick Count (ms)() -> (millisecond timer value=w320:u32)
                            n150 = Subtract(x=w320, y=w319) -> (x-y=w322:u32)
                            n151 = Divide(x=w322, y=u32 1000) -> (x/y=w317:dbl)
                            n152 = Build Array (concatenate)(w318, w317) -> (w316:dbl[])
                          }
                        }
                        n153 = local read "Start"() -> (w177:bool)
                      }
                    }
                    frame #1 {
                      # "set new Y\nand move to new position"
                      n154 = Increment(x=w334) -> (x+1=w333:i32)
                      n155 = local read "Start"() -> (w324:bool)
                      n156 = Equal?(x=w332, y=w333) -> (x = y?=w326:bool)
                      n157 = local read "Simulate Drive"() -> (w327:bool)
                      n158 = Not(x=w324) -> (.not. x?=w325:bool)
                      n159 = Or(x=w326, y=w325) -> (x .or. y?=w323:bool)
                      n160 = case shown="False" w323 {
                        tunnel: w330 -> [w355 w356]
                        tunnel: [w354 w356] -> w328
                        tunnel: w331 -> [w349 _]
                        frame False {
                          n161 = Unbundle By Name(w355) -> ("Drive Y Set"=w353:dbl)
                          n162 = Add(x=w349, y=w353) -> (x+y=w350:dbl)
                          n163 = Divide(x=w350, y=w349) -> (x/y=w351:dbl)
                          n164 = Round To Nearest(number=w351) -> (nearest integer value=w352:dbl)
                          n165 = Multiply(x=w352, y=w349) -> (x*y=w348:dbl)
                          n166 = Bundle By Name(cluster=w355, "Drive Y Set"=w348) -> (w354:T13)
                        }
                        frame True {
                        }
                      }
                      n167 = case shown="False" w327 {
                        tunnel: w329 -> [w338 _]
                        tunnel: w328 -> [w337 _]
                        frame False {
                          n168 = local read "Current Position"() -> (w336:T1)
                          n169 = Unbundle By Name(w336) -> ("Voltages.Drive Y Voltage"=w335:dbl)
                          n170 = flat-sequence {
                            tunnel: w338 -> [w341]
                            tunnel: w337 -> [w342]
                            tunnel: w335 -> [w343]
                            tunnel: [w341] -> w340
                            tunnel: [w347] -> w339
                            tunnel: w340 -> [w346]
                            frame #0 {
                              n171 = control-ref of="Objective Running"() -> (w345:refnum<vi>)
                              n172 = call "ESA-C Move Axis To.vi"("Drive Connection Settings"=w341, "Axis"=2, "Current Voltage (V)"=w343, "Drive New Abs. Positions"=w342, "Running"=w345) -> ()  [unwired: 2 in]
                            }
                            frame #1 {
                              n173 = call "ESA-C Get Values.vi"("Drive Connection Settings"=w346) -> ("Drive Current Values"=w347:T1)
                            }
                          }
                          n174 = local write "Current Position"(w339) -> ()
                        }
                        frame True {
                        }
                      }
                      n175 = local write "Target Position"(w328) -> ()
                    }
                  }
                  n176 = local read "Start"() -> (w120:bool)
                }
              }
              frame #2 {
                # "conclude measurement"
                n177 = flat-sequence {
                  tunnel: w358 -> [w363]
                  tunnel: w357 -> [w362]
                  tunnel: w359 -> [w386]
                  frame #0 {
                    # "save data"
                    n178 = local read "CCD3500 Temperature"() -> (w369:dbl)
                    n179 = local read "ITC503 Current Values"() -> (w371:T7)
                    n180 = local read "iHR Current Values"() -> (w370:T8)
                    n181 = local read "Mapping Params"() -> (w361:T5)
                    n182 = local read "Spectra Params"() -> (w366:T3)
                    n183 = Unbundle By Name(w361) -> ("Step Size"=w360:dbl)
                    n184 = local read "Live Data"() -> (w365:dbl[][])
                    n185 = call "Mapping Merge Real Positions v10.2.1.vi"("Live Data In"=w365, "X in (1D)"=w363, "Y in (1D)"=w362, "Step Size"=w360) -> ("Live Data Out"=w364:dbl[][])  [unwired: 11 in]
                    "Full Data" <- w364
                    n186 = call "Export_mappingFileName.vi"("ITC503 Current Values"=w371, "iHR Current Values"=w370, "Spectra Settings"=w366, "Mapping Parameters"=w361, "CCD3500 Temperature"=w369) -> ("Filename"=w367:string)
                    "Filename" <- w367
                    n187 = call "Export_2DtoTxt v10.2.0.vi"("Data (2D)"=w364, "Export Type"="Mapping", "Filename"=w367) -> ()  [unwired: 3 in]
                  }
                  frame #1 {
                    # "go to start"
                    n188 = local read "Drive Settings"() -> (w372:T4)
                    n189 = local read "Simulate Drive"() -> (w373:bool)
                    n190 = case shown="False" w373 {
                      tunnel: w372 -> [w375 _]
                      frame False {
                        n191 = stacked-sequence {
                          tunnel: w375 -> [w380 w384]
                          frame #0 {
                            n192 = local read "Mapping Params"() -> (w378:T5)
                            n193 = Unbundle By Name(w378) -> ("X Start Position"=w376:dbl, "Y Start Position"=w377:dbl)
                            n194 = local read "Target Position"() -> (w382:T2)
                            n195 = Bundle By Name(cluster=w382, "Drive X Set"=w376, "Drive Y Set"=w377) -> (w379:T2)
                            n196 = control-ref of="Objective Running"() -> (w381:refnum<vi>)
                            n197 = call "ESA-C Move Absolute.vi"("Running"=w381, "Drive New Abs. Positions"=w379, "Drive Connection Settings"=w380) -> ()  [unwired: 2 in]
                            n198 = local write "Target Position"(w379) -> ()
                          }
                          frame #1 {
                            n199 = call "ESA-C Get Values.vi"("Drive Connection Settings"=w384) -> ("Drive Current Values"=w383:T1)
                            n200 = local write "Current Position"(w383) -> ()
                          }
                        }
                        n201 = property on="Measuring" class="Bool (strict)"("BoolText.Text"="Homing...." ("Boolescher Text.Text")) -> ()  [unwired: 2 in, 2 out]
                      }
                      frame True {
                      }
                    }
                  }
                  frame #2 {
                    # "reset indicators"
                    n202 = case shown="False" w386 {
                      frame False {
                        n203 = call "Video Close.vi"() -> ()  [unwired: 11 in, 1 out]
                      }
                      frame True {
                      }
                    }
                    n204 = local write "Start"(FALSE ("Start")) -> ()
                    n205 = local write "CCD3000 Current Rep."("0/0" ("CCD3000 Current Rep.")) -> ()
                    n206 = property on="Measuring" class="Bool (strict)"("BoolText.Text"="" ("Boolescher Text.Text")) -> ()  [unwired: 2 in, 2 out]
                    n207 = property on="Measuring" class="Bool (strict)"("Blinking"=FALSE ("Measuring")) -> ()  [unwired: 2 in, 2 out]
                  }
                }
              }
            }
          }
        }
        n208 = local read "Exit"() -> (w34:bool)
      }
    }
    frame #2 {
      n209 = invoke class="VI Interface Type 0" method="Ctrl Val.Set"(reference=w390, "Control Name"="Exit" ("Elementname"), "Value"=TRUE) -> ()  [unwired: 2 in, 5 out]
      n210 = flat-sequence {
        frame #0 {
          # "return to center"
          n211 = local read "Simulate Drive"() -> (w393:bool)
          n212 = case shown="False" w393 {
            frame False {
              w399 = 10.0 ("Drive X Set")
              n213 = local read "Z Position"() -> (w398:dbl)
              n214 = local read "Target Position"() -> (w397:T2)
              n215 = local read "Drive Settings"() -> (w396:T4)
              n216 = Bundle By Name(cluster=w397, "Drive X Set"=w399, "Drive Y Set"=w399, "Drive Z Set"=w398) -> (w395:T2)
              n217 = control-ref of="Objective Running"() -> (w394:refnum<vi>)
              n218 = call "ESA-C Move Absolute.vi"("Running"=w394, "Drive New Abs. Positions"=w395, "Drive Connection Settings"=w396) -> ()  [unwired: 2 in]
            }
            frame True {
            }
          }
        }
        frame #1 {
          # "reset and close"
          n219 = control-ref of="Dieses VI"() -> (w400:refnum<vi>)
          n220 = invoke class="VI" method="Default Vals.Reinit All"(reference=w400) -> (reference out=w402:refnum<vi>)  [unwired: 2 in, 2 out]
          n221 = property on="Measuring" class="Bool (strict)"("BoolText.Text"="" ("Boolescher Text.Text")) -> ()  [unwired: 2 in, 2 out]
          n222 = property class="App"() -> ("App.Kind"=w401:T16)  [unwired: 2 in, 2 out]
          n223 = case shown="\"Development System\"" w401 {
            tunnel: w402 -> [w404 _]
            frame "invalid app kind", Default {
              n224 = invoke on="Invoke Node" class="VI" method="FP.Close"(reference=w404) -> ()  [unwired: 2 in, 3 out]
            }
            frame "Development System" {
            }
          }
        }
      }
    }
  }
